vi "CreateSelectString.vi"(7 "# of row (90)":i32=90, 10 "Items":string[](array[string])=["C1", "C2", "C3"], 11 "Table Name":string="temp") -> (3 "Create Select String (by Time)":string)   [LabVIEW 2015, in "DBToolkit.lvlib"]
uses:
  DBToolkit.lvlib
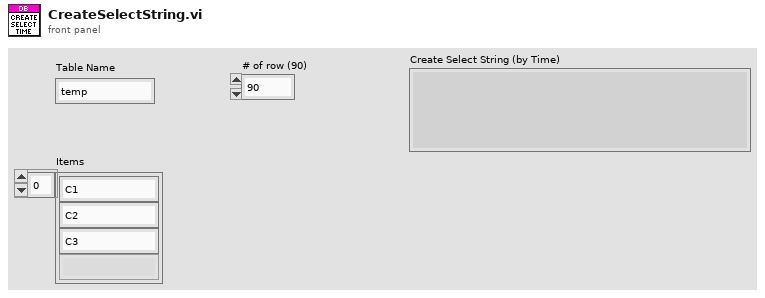
[diagram p1: front panel]
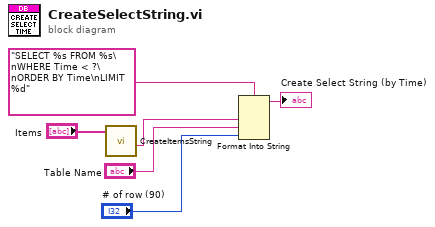
[diagram p0: block diagram]
diagram:
  n1 = call "CreateItemsString.vi"("Items"="Items") -> ("Items for SELECT"=w3:string)  [unwired: 8 in, 2 out]
  n2 = Format Into String(format string="SELECT %s FROM %s\nWHERE Time < ?\nORDER BY Time\nLIMIT %d", w3, "Table Name", "# of row (90)") -> (resulting string=→"Create Select String (by Time)":string)  [unwired: 2 in, 1 out]
